vi "MouseMoveTrackingSwitch.vi"(9 "State":enum16{"Stop", "Start"}(ring), 10 "Controls Reference In":T1, 11 "Event Registration Refnum In":refnum<event-registration>) -> (3 "Event Registration Refnum Out":refnum<event-registration>)   [LabVIEW 2017]
uses:
  TypeDefinitions/ExperimentControls.ctl
  AODControl/AODControlFiles/InterfaceReferences.ctl
  AODControl/AODControlFiles/LoadControl.ctl
  AODControl/AODControlFiles/ExitButton.ctl
  ImageAcquisitionProgram/ImageAcquisitionLibrary/References.ctl
  AODControl/AODControl.lvlib
  ImageAcquisitionProgram/ImageAcquisitionLibrary/ImageAcquisitionLibrary.lvlib
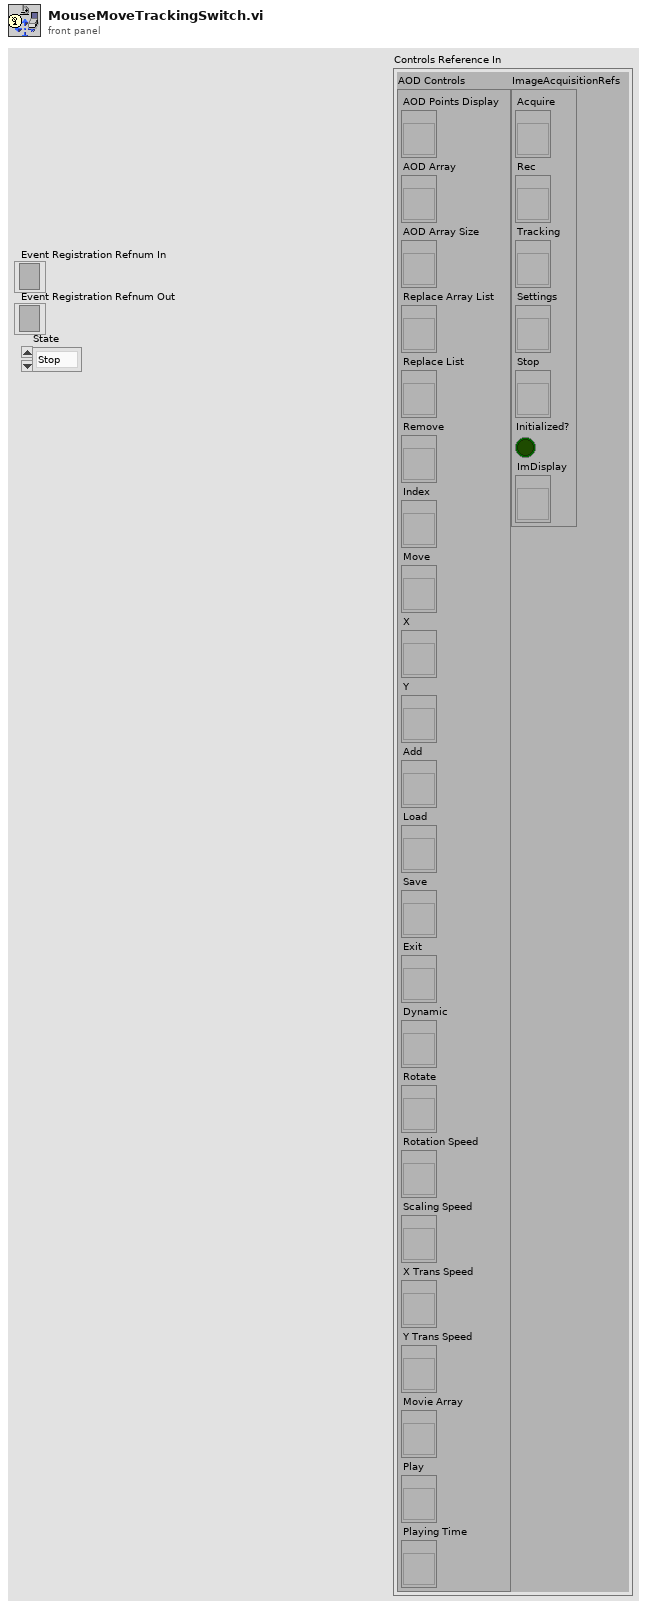
[diagram p1: front panel]
types:
  T1 = typedef "ExperimentControls.ctl" = cluster{"AOD Controls":T2, "ImageAcquisitionRefs":T3}
  T2 = typedef "AODControl.lvlib/InterfaceReferences.ctl" = cluster{"AOD Points Display":refnum<vi>, "AOD Array":refnum<vi>, "AOD Array Size":refnum<vi>, "Replace Array List":refnum<vi>, "Replace List":refnum<vi>, "Remove":refnum<vi>, "Index":refnum<vi>, "Move":refnum<vi>, "X":refnum<vi>, "Y":refnum<vi>, "Add":refnum<vi>, "Load":refnum<vi>, "Save":refnum<vi>, "Exit":refnum<vi>, "Dynamic":refnum<vi>, "Rotate":refnum<vi>, "Rotation Speed":refnum<vi>, "Scaling Speed":refnum<vi>, "X Trans Speed":refnum<vi>, "Y Trans Speed":refnum<vi>, "Movie Array":refnum<vi>, "Play":refnum<vi>, "Playing Time":refnum<vi>}
  T3 = typedef "ImageAcquisitionLibrary.lvlib/References.ctl" = cluster{"Acquire":refnum<vi>, "Rec":refnum<vi>, "Tracking":refnum<vi>, "Settings":refnum<vi>, "Stop":refnum<vi>, "Initialized?":bool, "ImDisplay":refnum<vi>}
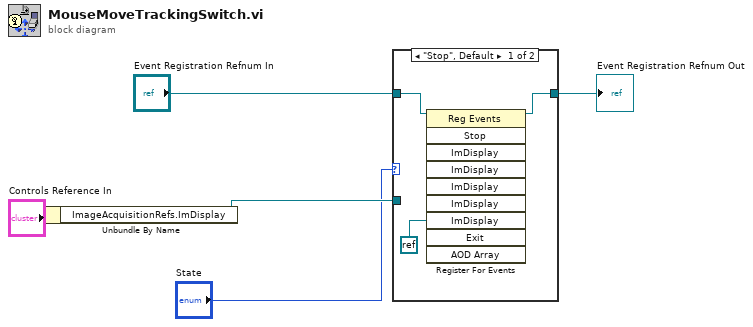
[diagram p0: block diagram]
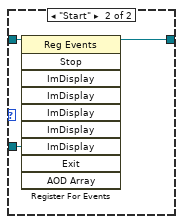
[diagram p2: hidden frame]
diagram:
  n1 = Unbundle By Name("Controls Reference In") -> ("ImageAcquisitionRefs.ImDisplay"=w2:refnum<vi>)
  n2 = case shown="\"Stop\", Default" "State" {
    tunnel: [w7 w11] -> w5
    tunnel: "Event Registration Refnum In" -> [w8 w10]
    tunnel: w2 -> [_ w9]
    frame "Stop", Default {
      n3 = register-events(reference=w8, refnum<k0> refnum) -> (reference out=w7:refnum<event-registration>)  [unwired: 8 in, 1 out]
    }
    frame "Start" {
      n4 = register-events(reference=w10, w9) -> (reference out=w11:refnum<event-registration>)  [unwired: 8 in, 1 out]
    }
  }
  "Event Registration Refnum Out" <- w5
